vi "Turn On Off Circulator.vi"(6 "Initialize/Close?":bool, 8 "Error In (No Error)":errorcluster, 9 "Circulator On/Off":bool, 10 "Sensor Address In":string="0", 11 "RS232 Port In":refnum<visa-resource-name>="COM11") -> (0 "Error Out":errorcluster, 1 "Circulator On/Off Response":bool, 2 "Address Out":string, 3 "RS232 Port Out":refnum<visa-resource-name>)   [LabVIEW 2016]
doc: "Sends an SDI-12 Send Identification Command, and returns the various attributes from the sensor's response.\n\nThe total size by the sensor must be 22-35 in size (inclusive), or this VI will return an error."
uses:
  SDI-12/SDI-12.lvlib
panel:
  out "read buffer":string
  out "output 1":i16
  out "Command":string
  # "(c) 2008 National Instruments.  ALL RIGHTS RESERVED."
  # "The following are required,\nor are optional, for the sensors\nto respond with:"
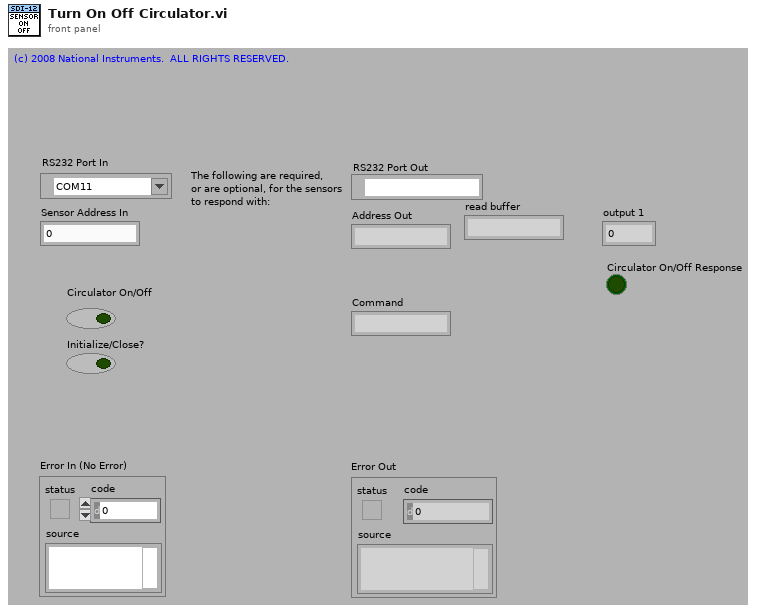
[diagram p1: front panel]
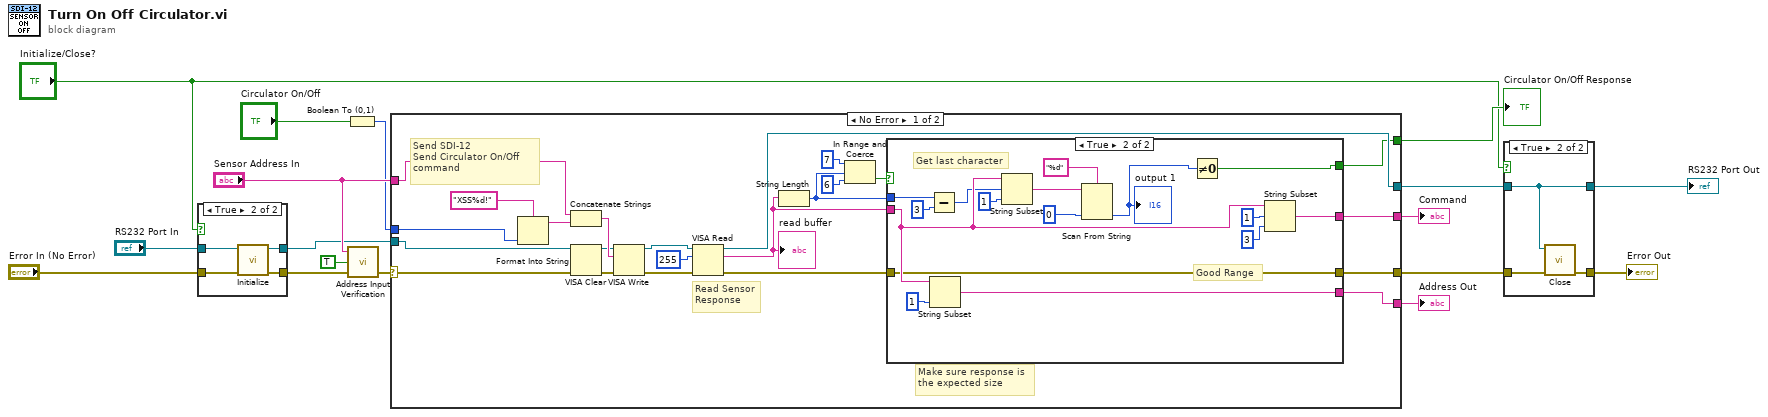
[diagram p0: block diagram]
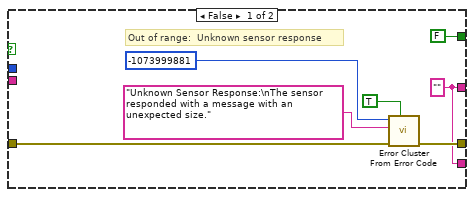
[diagram p4: hidden frame]
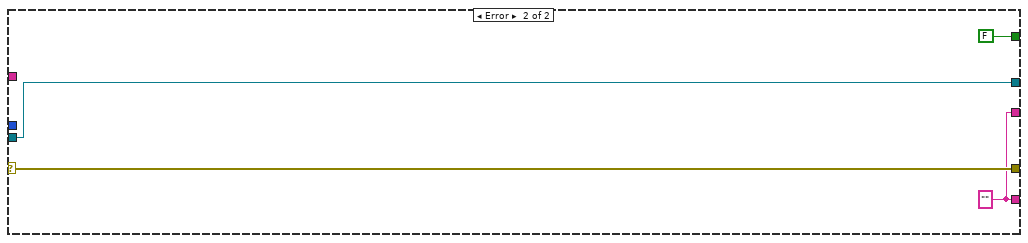
[diagram p5: hidden frame]
diagram:
  n1 = case shown="True" "Initialize/Close?" {
    tunnel: "Error In (No Error)" -> [w19 w23]
    tunnel: [w19 w22] -> w2
    tunnel: "RS232 Port In" -> [w18 w21]
    tunnel: [w18 w20] -> w5
    frame False {
    }
    frame True {
      n2 = call "Initialize.vi"("Error In (No Error)"=w23, "RS232 Port In"=w21) -> ("Error Out"=w22:errorcluster, "RS232 Port Out"=w20:refnum<visa-resource-name>)  [unwired: 8 in]
    }
  }
  n3 = Boolean To (0,1)(Boolean="Circulator On/Off") -> (0, 1=w11:i16)
  n4 = call "Address Input Verification.vi"("Error In (No Error)"=w2, "Error if Bad? (True)"=TRUE ("error if bad? (True)"), "Sensor Address In (a)"="Sensor Address In") -> ("Error Out"=w17:errorcluster)  [unwired: 1 in, 1 out]
  n5 = case shown="No Error" w17 {
    selector: w17 -> [w26 w73]
    tunnel: [w34 w73] -> w7
    tunnel: "Sensor Address In" -> [w43 _]
    tunnel: w5 -> [w41 w72]
    tunnel: [w40 w72] -> w6
    tunnel: [w33 w71] -> w13
    tunnel: [w32 w71] -> w14
    tunnel: w11 -> [w31 _]
    tunnel: [w28 FALSE] -> w10
    frame No Error {
      # "Make sure response is\nthe expected size"
      # "Send SDI-12 \nSend Circulator On/Off \ncommand"
      # "Read Sensor\nResponse"
      n6 = Format Into String(format string="XSS%d!", w31) -> (resulting string=w29:string)  [unwired: 2 in, 1 out]
      n7 = Concatenate Strings(w43, w29) -> (w42:string)
      n8 = VISA Clear(VISA resource name=w41, error in (no error)=w26) -> (VISA resource name out=w27:refnum<visa-resource-name>, error out=w25:errorcluster)
      n9 = VISA Write(VISA resource name=w27, write buffer=w42, error in (no error)=w25) -> (VISA resource name out=w46:refnum<visa-resource-name>, error out=w45:errorcluster)  [unwired: 1 out]
      n10 = VISA Read(VISA resource name=w46, byte count=u32 255, error in (no error)=w45) -> (VISA resource name out=w40:refnum<visa-resource-name>, read buffer=w36:string, error out=w37:errorcluster)  [unwired: 1 out]
      "read buffer" <- w36
      n11 = String Length(string=w36) -> (length=w24:i32)
      n12 = In Range and Coerce(upper limit=7, x=w24, lower limit=6) -> (In Range?=w35:bool)  [unwired: 1 out]
      n13 = case shown="True" w35 {
        tunnel: w37 -> [w49 w64]
        tunnel: [w50 w64] -> w34
        tunnel: w36 -> [_ w66]
        tunnel: [w48 w62] -> w33
        tunnel: [w48 w61] -> w32
        tunnel: [FALSE w57] -> w28
        tunnel: w24 -> [_ w56]
        frame False {
          w48 = "" ("read buffer")
          # "Out of range:  Unknown sensor response"
          n14 = call <vilib>:"Error Cluster From Error Code.vi"("show call chain? (False)"=TRUE, "error in (no error)"=w49, "error message (\"\")"="Unknown Sensor Response:\nThe sensor responded with a message with an unexpected size." ("error message (\"\")"), "error code (0)"=-1073999881) -> ("error out"=w50:errorcluster)  [unwired: 5 in]
        }
        frame True {
          # "Get last character"
          # "Good Range"
          n15 = Subtract(x=w56, y=3) -> (x-y=w54:i32)
          n16 = String Subset(string=w66, length (rest)=1 ("length (rest)")) -> (substring=w61:string)  [unwired: 1 in]
          n17 = String Subset(string=w66, offset (0)=w54, length (rest)=1 ("length (rest)")) -> (substring=w63:string)
          n18 = Scan From String(format string="%d", input string=w63, default 1=i16 0 ("default value 1")) -> (output 1=w58:i16)  [unwired: 2 in, 3 out]
          "output 1" <- w58
          n19 = Not Equal To 0?(x=w58) -> (x != 0?=w57:bool)
          n20 = String Subset(string=w66, offset (0)=1, length (rest)=3 ("length (rest)")) -> (substring=w62:string)
        }
      }
    }
    frame Error {
      w71 = "" ("read buffer")
    }
  }
  "Command" <- w13
  "Address Out" <- w14
  "Circulator On/Off Response" <- w10
  n21 = case shown="True" "Initialize/Close?" {
    tunnel: w7 -> [w75 w78]
    tunnel: [w75 w77] -> w8
    tunnel: w6 -> [w74 w76]
    tunnel: [w74 w76] -> w9
    frame False {
    }
    frame True {
      n22 = call "Close.vi"("Error In (No Error)"=w78, "RS232 Port In"=w76) -> ("Error Out"=w77:errorcluster)  [unwired: 9 in]
    }
  }
  "Error Out" <- w8
  "RS232 Port Out" <- w9
